vi "LVClass_HasoEngine Read HasoSlopes.vi"(8 "error in (no error)":errorcluster, 11 "HasoEngine in":refnum<class "HasoEngine.lvclass">) -> (0 "error out":errorcluster, 2 "HasoSlopes.lvclass":refnum<class "HasoSlopes.lvclass">, 3 "HasoEngine out":refnum<class "HasoEngine.lvclass">)   [LabVIEW 2020, in "HasoEngine.lvclass"]
uses:
  HasoEngine.lvclass
  HasoSlopes.lvclass
  HasoEngine.lvclass/HasoEngine.ctl
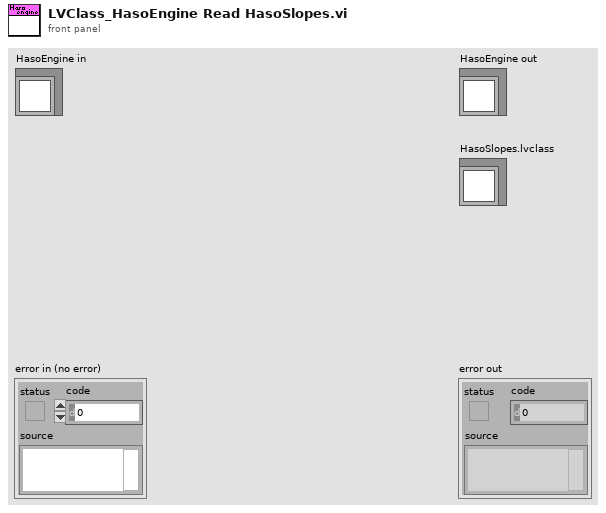
[diagram p1: front panel]
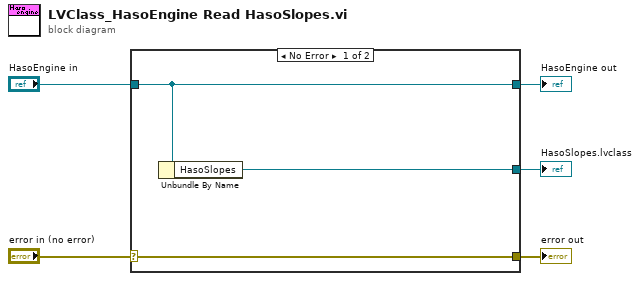
[diagram p0: block diagram]
diagram:
  n1 = case shown="No Error" "error in (no error)" {
    selector: "error in (no error)" -> [w8 w9]
    tunnel: [w8 w9] -> w4
    tunnel: [w7 w10] -> w2
    tunnel: "HasoEngine in" -> [w7 w10]
    tunnel: [w6 _] -> w1
    frame No Error {
      n2 = Unbundle By Name(w7) -> ("HasoSlopes"=w6:refnum<class "HasoSlopes.lvclass">)
    }
    frame Error {
    }
  }
  "error out" <- w4
  "HasoEngine out" <- w2
  "HasoSlopes.lvclass" <- w1
